vi "Create Shared Variables for All Channels.vi"(8 "error in":errorcluster) -> (0 "error out":errorcluster, 2 "Variable Names":string[](array[string]))   [LabVIEW 2017, in "DTACQ - Network Enabled Device Driver.lvlib"]
uses:
  DTACQ - Network Enabled Device Driver.lvlib
  Communications/Typedefs/DTACQ Device Type--Enum.ctl
  Network Shared Variables/Typedefs/X and Y Variant Arrays--Cluster.ctl
  Communications/Communications Library.lvlib
  Network Shared Variables/Shared Variables Library.lvlib
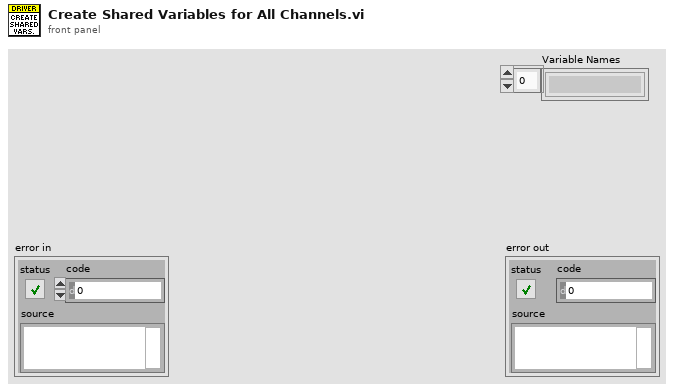
[diagram p1: front panel]
types:
  T1 = typedef "Shared Variables Library.lvlib/X and Y Variant Arrays--Cluster.ctl" = cluster{"X-Data":variant[], "Y-Data":variant[]}
  T2 = typedef "Communications Library.lvlib/DTACQ Device Type--Enum.ctl" = enum16{"Carrier", "Analog In Module", "Analog Out Module", "Generic Module"}
  T3 = typedef "Communications Library.lvlib/DTACQ Module Configuration--Cluster.ctl" = cluster{"Name":string, "Position":string, "Module Type":T2, "Control Port":i32, "Timeout (ms)":i32, "Channels":i32}
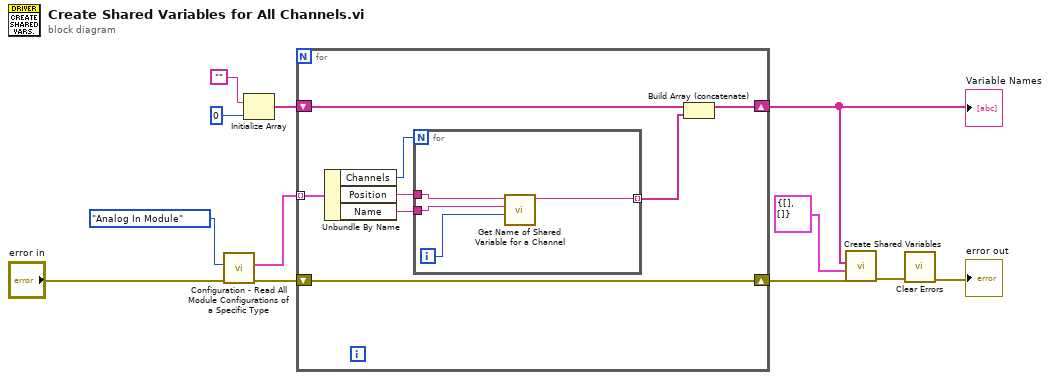
[diagram p0: block diagram]
diagram:
  n1 = call "Configuration - Read All Module Configurations of a Specific Type.vi"("error in"="error in", "Module Type"=DTACQ_Device_Type--Enum."Analog In Module") -> ("error out"=w10:errorcluster, "Module Configurations"=w11:T3[])  [unwired: 7 in, 1 out]
  n2 = Initialize Array("", 0) -> (w6:string[])
  n3 = for {
    tunnel: w11 -> [w20] mode=indexing
    shift-right: [w17] -> w9
    shift-left: w10 -> [w17]
    shift-right: [w13] -> w5
    shift-left: w6 -> [w15]
    n4 = Unbundle By Name(w20) -> ("Channels"=w16:i32, "Position"=w19:string, "Name"=w18:string)
    n5 = for {
      N: w16 -> [_]
      tunnel: w19 -> [w24]
      tunnel: w18 -> [w23]
      tunnel: [w22] -> w14 mode=indexing
      i -> [w21]
      n6 = call "Get Name of Shared Variable for a Channel.vi"("Channel Number"=w21, "Module Name"=w23, "Module Position"=w24) -> ("Shared Variable Name"=w22:string)  [unwired: 8 in]
    }
    n7 = Build Array (concatenate)(w15, w14) -> (w13:string[])
  }
  "Variable Names" <- w5
  n8 = call "Create Shared Variables.vi"("error in"=w9, "Data Type"=T1 {"X-Data"=[], "Y-Data"=[]} ("Data Cluster"), "Variable Names"=w5) -> ("error out"=w4:errorcluster)  [unwired: 8 in]
  n9 = call <vilib>:"Clear Errors.vi"("error in (no error)"=w4) -> ("error out"=→"error out":errorcluster)  [unwired: 5 in, 1 out]
